vi "LVDimInterface.dis_update_service.vi"(0 "my_serviceID":i32, 2 "data":string, 5 "error in (no error)":errorcluster) -> (14 "my_serviceID out":i32, 15 "nOfClients":i32, 19 "error out":errorcluster)   [LabVIEW 2014, in "LVDimInterface.lvlib"]
doc: "This routine should be called by the server program when there is a change for a given service (when possible). This routine will check whether there are clients interested in this service and if they have requested to receive the data upon change (monitored service) the data will be sent by sending the specified data buffer.\n\n\nHistory: 16-DEC-2005, Dietrich Beck\n\nCopyright (C)\nGesellschaft für Schwerionenforschung, GSI\nPlanckstr. 1\n64291 Darmstadt\nGermany\n\nContact: D.Beck@gsi.de \n\nThis program is free software; you can redistribute it and/or modify it under the terms of the \nGNU General Public License as published by the Free Software Foundation; either version 2 of the license, or (at your option) any later version.\n\nThis program is distributed in the hope that it will be useful, but WITHOUT ANY WARRANTY; without even the implied warranty of MERCHANTABILITY or FITNESS FOR A PARTICULAR PURPOSE. See the GNU General License for more details (http://www.gnu.org).\n\nGesellschaft für Schwerionenforschung, GSI\nPlanckstr. 1, 64291 Darmstadt, Germany\nFor all questions and ideas contact D. Beck.\nLast update: 16-DEC-2005"
uses:
  LVDimInterface.lvlib
  shs/packages/dmdriver/DMirrorPCS/libDimWrapper.dll
  bin/libDimWrapper.so
  bin/libDimWrapperSPL.dll
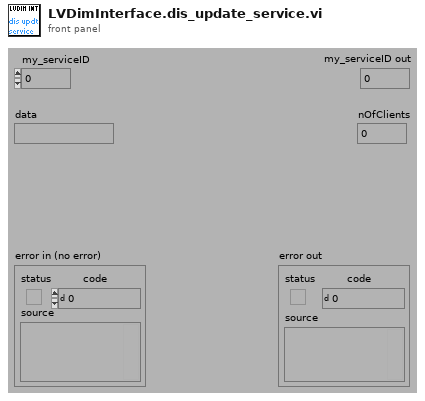
[diagram p1: front panel]
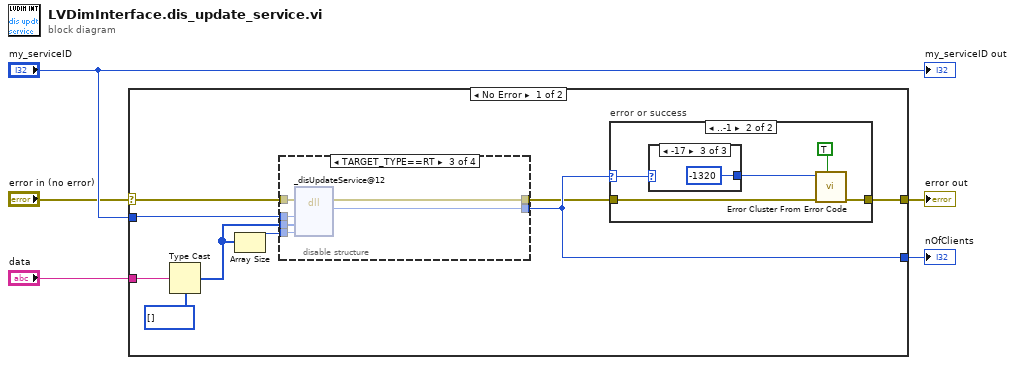
[diagram p0: block diagram]
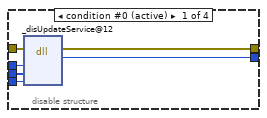
[diagram p2: hidden frame]
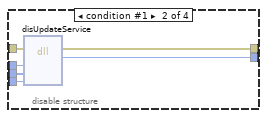
[diagram p3: hidden frame]
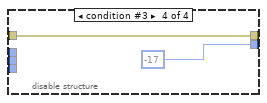
[diagram p4: hidden frame]
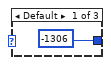
[diagram p6: hidden frame]
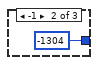
[diagram p7: hidden frame]
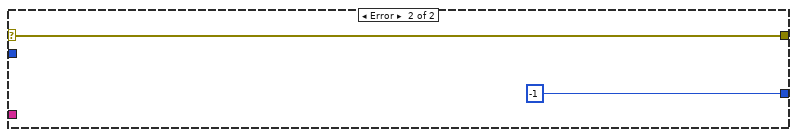
[diagram p8: hidden frame]
diagram:
  n1 = case shown="No Error" "error in (no error)" {
    selector: "error in (no error)" -> [w7 w44]
    tunnel: [w14 -1 ("nOfClients")] -> w5
    tunnel: [w12 w44] -> w4
    tunnel: "my_serviceID" -> [w13 _]
    tunnel: "data" -> [w11 _]
    frame No Error {
      n2 = Type Cast(type=i8[] [], x=w11) -> (*(type *) &x=w10:i8[])
      n3 = Array Size(array=w10) -> (size(s)=w8:i32)
      n4 = disable-structure "Conditional Disable Structure" shown="TARGET_TYPE==RT" {
        disable-tunnel: [w20 w26 w32 -17 ("nOfClients")] -> w14
        disable-tunnel: w13 -> [w19 w25 w31 _]
        disable-tunnel: w8 -> [w18 w24 w30 _]
        disable-tunnel: w10 -> [w17 w23 w29 _]
        disable-tunnel: w7 -> [w16 w22 w28 w33]
        disable-tunnel: [w15 w21 w27 w33] -> w6
        frame condition #0 (active) {
          n5 = dll-call lib="D:/Git/CS-framework/CSlibraries-extern/shs/packages/dmdriver/DMirrorPCS/libDimWrapper.dll" fn="_disUpdateService@12" label="disUpdateService"(error in=w16, "my_serviceID"=w19, "data"=w17, "size"=w18) -> (error out=w15:errorcluster, "nOfClients"=w20:i32)  [unwired: 5 in, 1 out]
        }
        frame condition #1 {
          n6 = dll-call lib="D:/Git/CS-framework/CSlibraries/DimLVEvent/bin/libDimWrapper.so" fn="disUpdateService"(error in=w22, "my_serviceID"=w25, "data"=w23, "size"=w24) -> (error out=w21:errorcluster, "nOfClients"=w26:i32)  [unwired: 5 in, 1 out]
        }
        frame condition #2 {
          n7 = dll-call lib="D:/Git/CS-framework/CSlibraries/DimLVEvent/bin/libDimWrapperSPL.dll" fn="_disUpdateService@12" label="libDimWrapper.so:disUpdateService"(error in=w28, "my_serviceID"=w31, "data"=w29, "size"=w30) -> (error out=w27:errorcluster, "nOfClients"=w32:i32)  [unwired: 5 in, 1 out]
        }
        frame condition #3 {
        }
      }
      n8 = case "error or success" shown="..-1" w14 {
        selector: w14 -> [_ w40]
        tunnel: w6 -> [w35 w38]
        tunnel: [w35 w39] -> w12
        frame 0, Default {
        }
        frame ..-1 {
          n9 = case shown="-17" w40 {
            tunnel: [-1306 ("f") -1304 ("code") -1320 ("code")] -> w37
            frame Default {
            }
            frame -1 {
            }
            frame -17 {
            }
          }
          n10 = call <vilib>:"Error Cluster From Error Code.vi"("show call chain? (False)"=TRUE, "error in (no error)"=w38, "error code (0)"=w37) -> ("error out"=w39:errorcluster)  [unwired: 6 in]
        }
      }
    }
    frame Error {
    }
  }
  "error out" <- w4
  "nOfClients" <- w5
  "my_serviceID out" <- "my_serviceID"
